vi "Z-trial.vi"() -> ()   [LabVIEW 2010]
panel:
  out "slice number":i32
  out "GetPositionOffset 2":i32
  out "pfPosOffset 2":sgl
  out "pfPosOffset":sgl
  out "GetPositionOffset":i32
  out "pfAbsPos 2":sgl
  out "pfAbsPos":sgl
  out "fAbsPos":sgl
  in  "desired position":dbl
  out "Actual Z position 3":sgl
  in  "move Z absolute value":bool
  out "Actual Z position 2":sgl
  out "GetPosition 2":i32
  in  "get Z":bool
  in  "scan z":bool
  in  "number of slices":i32
  out "Actual Z position":sgl
  out "GetPosition":i32
  out "Cal. Z":dbl
  in  "Z Step Size":dbl
  in  "Starting Z  Position":dbl
  in  "Z scanner":refnum<k7>(container)
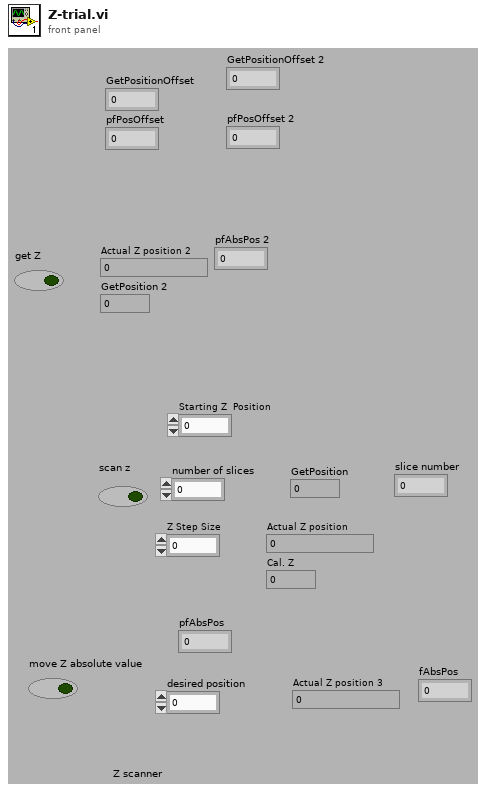
[diagram p1: front panel]
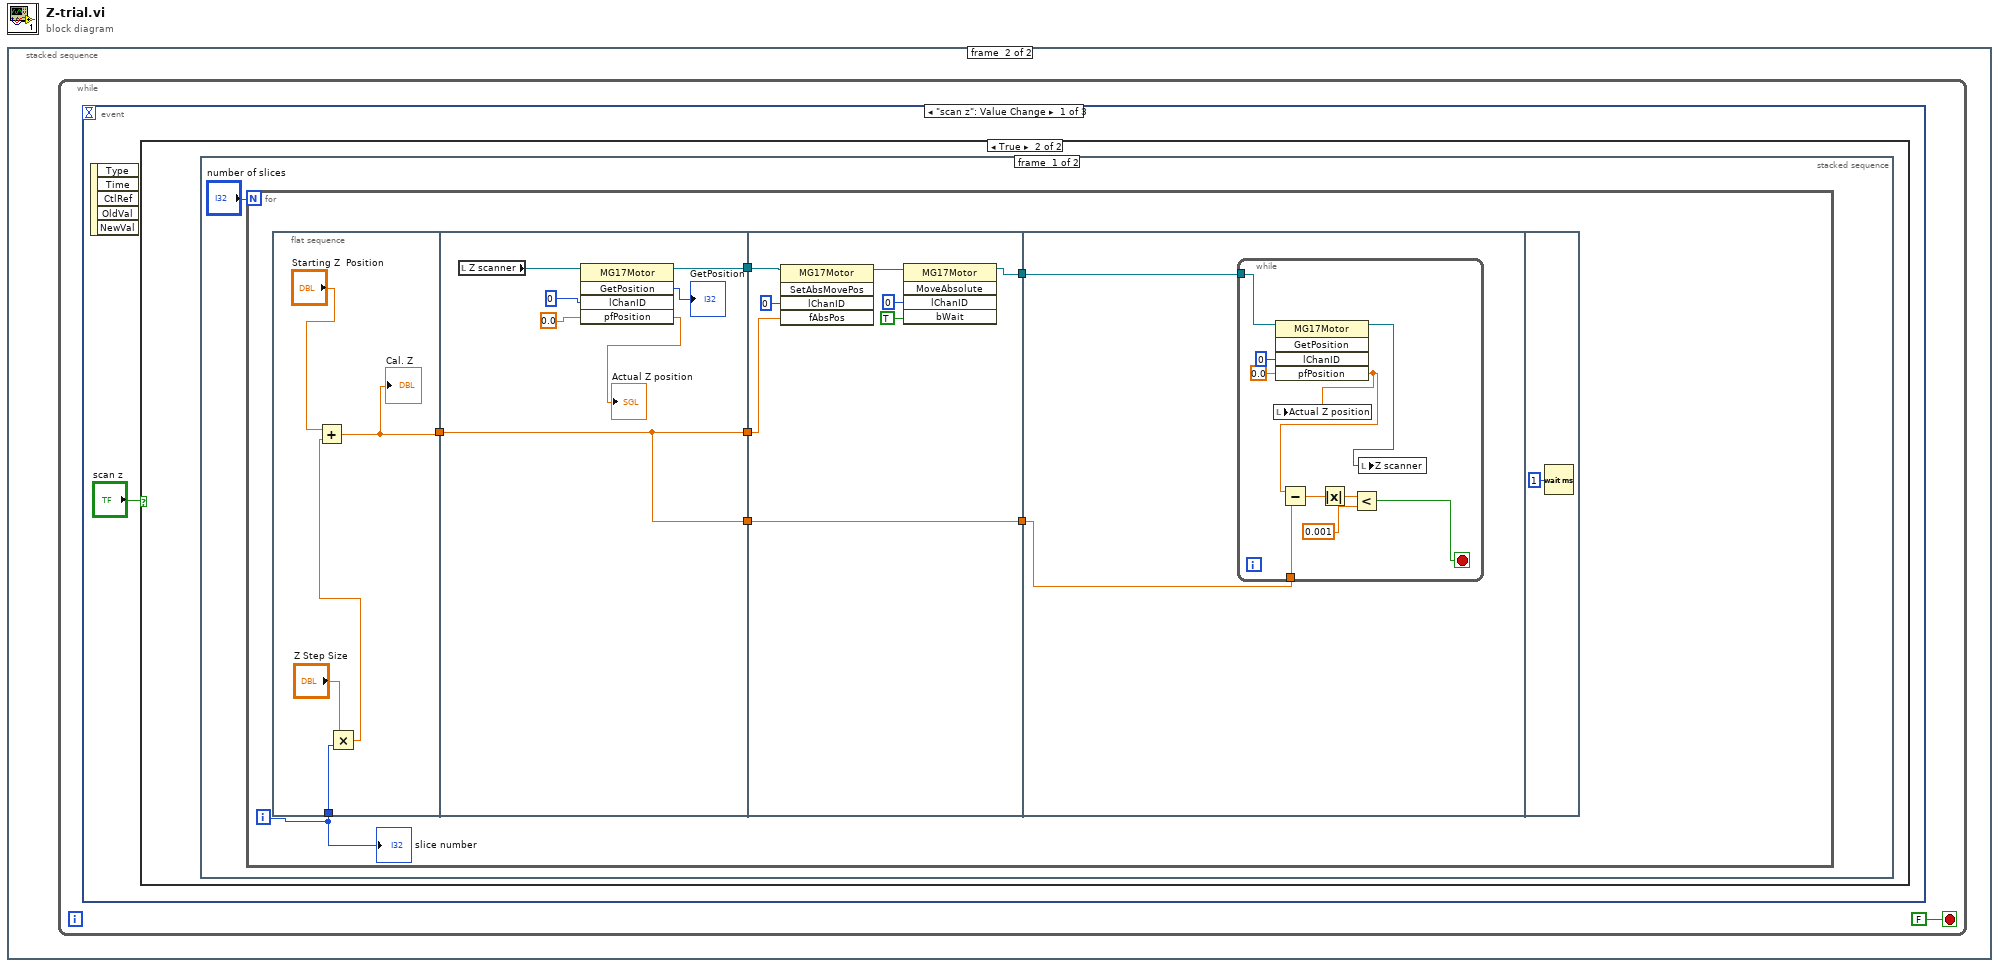
[diagram p0: block diagram]
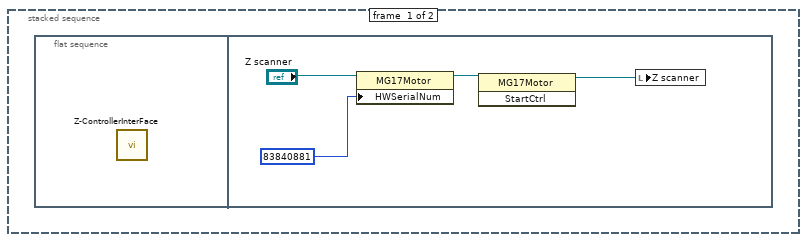
[diagram p2: hidden frame]
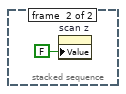
[diagram p4: hidden frame]
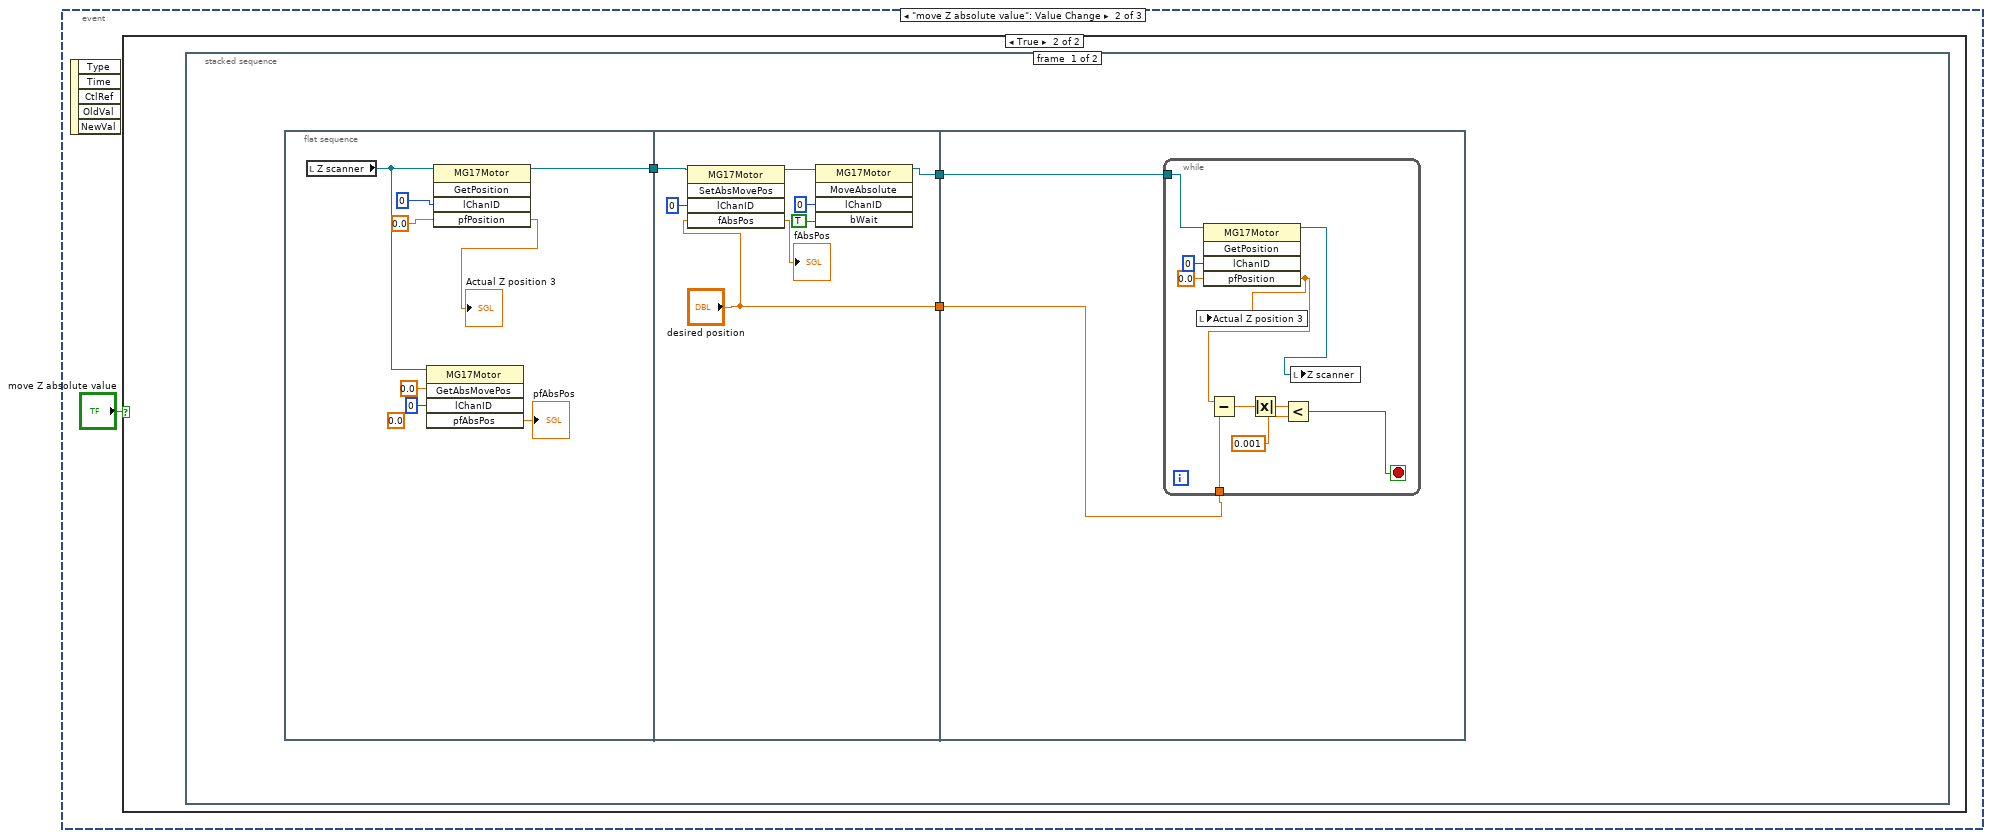
[diagram p5: hidden frame]
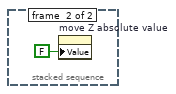
[diagram p7: hidden frame]
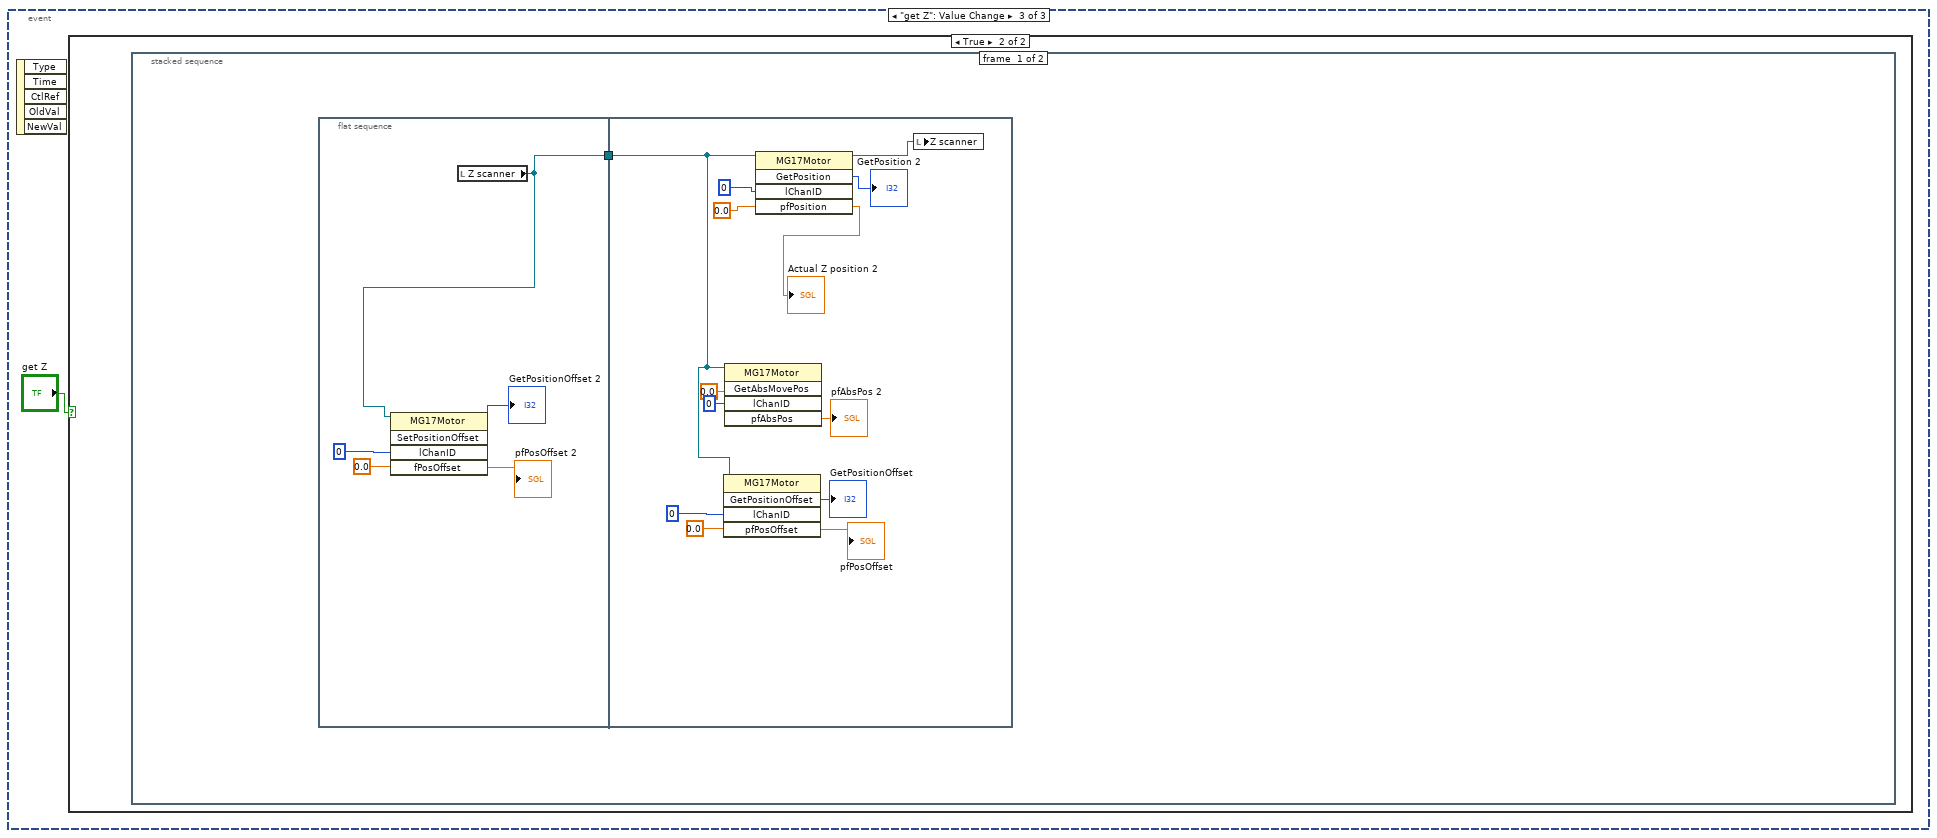
[diagram p8: hidden frame]
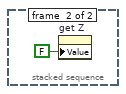
[diagram p10: hidden frame]
diagram:
  n1 = stacked-sequence {
    frame #0 {
      n2 = flat-sequence {
        frame #0 {
          n3 = call "Z-ControllerInterFace.vi"() -> ()  [unwired: 12 in]
        }
        frame #1 {
          n4 = property class="MG17Motor"(reference="Z scanner", "HWSerialNum"=83840881) -> (reference out=w3:refnum<k7>)  [unwired: 1 in, 1 out]
          n5 = invoke class="MG17Motor" method="StartCtrl"(reference=w3) -> (reference out=w1:refnum<k7>)  [unwired: 2 in, 2 out]
          n6 = local write "Z scanner"(w1) -> ()
        }
      }
    }
    frame #1 {
      n7 = while {
        stop <- FALSE stop-if-true
        n8 = event shown="[0] \"scan z\": Value Change" {
          selector: _ -> [_ _ _]
          dyn-events: _ -> [_ _ _]
          timeout: _ -> [_ _ _]
          event "scan z": Value Change {
            n9 = event-data() -> ()  [unwired: 1 in, 5 out]
            n10 = case shown="True" "scan z" {
              frame False {
              }
              frame True {
                n11 = stacked-sequence {
                  frame #0 {
                    n12 = for {
                      N: "number of slices" -> [_]
                      i -> [w8]
                      n13 = flat-sequence {
                        tunnel: [w18] -> w14
                        tunnel: w8 -> [w15]
                        tunnel: [w24] -> w13
                        tunnel: w14 -> [w23]
                        tunnel: [w23] -> w12
                        tunnel: [w23] -> w11
                        tunnel: w13 -> [w34]
                        tunnel: w12 -> [w32]
                        tunnel: w11 -> [w28]
                        tunnel: [w28] -> w10
                        tunnel: [w27] -> w9
                        tunnel: w10 -> [w36]
                        tunnel: w9 -> [w35]
                        frame #0 {
                          n14 = Multiply(x="Z Step Size", y=w15) -> (x*y=w19:dbl)
                          n15 = Add(x="Starting Z  Position", y=w19) -> (x+y=w18:dbl)
                          "Cal. Z" <- w18
                        }
                        frame #1 {
                          n16 = local read "Z scanner"() -> (w22:refnum<k7>)
                          n17 = invoke class="MG17Motor" method="GetPosition"(reference=w22, "lChanID"=0, "pfPosition"=sgl 0.0) -> (reference out=w24:refnum<k7>, "GetPosition"=→"GetPosition":i32, "pfPosition"=→"Actual Z position":sgl)  [unwired: 2 in, 2 out]
                        }
                        frame #2 {
                          n18 = invoke class="MG17Motor" method="SetAbsMovePos"(reference=w34, "lChanID"=0, "fAbsPos"=w32) -> (reference out=w33:refnum<k7>)  [unwired: 2 in, 4 out]
                          n19 = invoke class="MG17Motor" method="MoveAbsolute"(reference=w33, "lChanID"=0, "bWait"=TRUE) -> (reference out=w27:refnum<k7>)  [unwired: 2 in, 4 out]
                        }
                        frame #3 {
                          n20 = while {
                            tunnel: w36 -> [w43]
                            tunnel: w35 -> [w38]
                            stop <- w39 stop-if-true
                            n21 = invoke class="MG17Motor" method="GetPosition"(reference=w38, "lChanID"=0, "pfPosition"=sgl 0.0) -> (reference out=w37:refnum<k7>, "pfPosition"=w44:sgl)  [unwired: 2 in, 3 out]
                            n22 = local write "Actual Z position"(w44) -> ()
                            n23 = Subtract(x=w44, y=w43) -> (x-y=w42:dbl)
                            n24 = Absolute Value(x=w42) -> (abs(x)=w41:dbl)
                            n25 = Less?(x=w41, y=0.001) -> (x < y?=w39:bool)
                            n26 = local write "Z scanner"(w37) -> ()
                          }
                        }
                        frame #4 {
                          n27 = Wait (ms)(milliseconds to wait=u32 1) -> ()  [unwired: 1 out]
                        }
                      }
                      "slice number" <- w8
                    }
                  }
                  frame #1 {
                    n28 = property on="scan z" class="Bool (strict)"("Value"=FALSE ("scan z")) -> ()  [unwired: 2 in, 2 out]
                  }
                }
              }
            }
          }
          event "move Z absolute value": Value Change {
            n29 = event-data() -> ()  [unwired: 1 in, 5 out]
            n30 = case shown="True" "move Z absolute value" {
              frame False {
              }
              frame True {
                n31 = stacked-sequence {
                  frame #0 {
                    n32 = flat-sequence {
                      tunnel: [w58] -> w52
                      tunnel: w52 -> [w68]
                      tunnel: [w63] -> w51
                      tunnel: ["desired position"] -> w50
                      tunnel: w51 -> [w70]
                      tunnel: w50 -> [w69]
                      frame #0 {
                        (unwired) sgl 0.0 ("pfAbsPos")
                        n33 = local read "Z scanner"() -> (w56:refnum<k7>)
                        n34 = invoke class="MG17Motor" method="GetAbsMovePos"(reference=w56, "lChanID"=0, "pfAbsPos"=sgl 0.0) -> ("pfAbsPos"=→"pfAbsPos":sgl)  [unwired: 2 in, 4 out]
                        n35 = invoke class="MG17Motor" method="GetPosition"(reference=w56, "lChanID"=0, "pfPosition"=sgl 0.0) -> (reference out=w58:refnum<k7>, "pfPosition"=→"Actual Z position 3":sgl)  [unwired: 2 in, 3 out]
                      }
                      frame #1 {
                        n36 = invoke class="MG17Motor" method="SetAbsMovePos"(reference=w68, "lChanID"=0, "fAbsPos"="desired position") -> (reference out=w67:refnum<k7>, "fAbsPos"=→"fAbsPos":sgl)  [unwired: 2 in, 3 out]
                        n37 = invoke class="MG17Motor" method="MoveAbsolute"(reference=w67, "lChanID"=0, "bWait"=TRUE) -> (reference out=w63:refnum<k7>)  [unwired: 2 in, 4 out]
                      }
                      frame #2 {
                        n38 = while {
                          tunnel: w69 -> [w77]
                          tunnel: w70 -> [w72]
                          stop <- w73 stop-if-true
                          n39 = invoke class="MG17Motor" method="GetPosition"(reference=w72, "lChanID"=0, "pfPosition"=sgl 0.0) -> (reference out=w71:refnum<k7>, "pfPosition"=w78:sgl)  [unwired: 2 in, 3 out]
                          n40 = local write "Actual Z position 3"(w78) -> ()
                          n41 = Subtract(x=w78, y=w77) -> (x-y=w76:dbl)
                          n42 = Absolute Value(x=w76) -> (abs(x)=w75:dbl)
                          n43 = Less?(x=w75, y=0.001) -> (x < y?=w73:bool)
                          n44 = local write "Z scanner"(w71) -> ()
                        }
                      }
                    }
                  }
                  frame #1 {
                    n45 = property on="move Z absolute value" class="Bool (strict)"("Value"=FALSE ("scan z")) -> ()  [unwired: 2 in, 2 out]
                  }
                }
              }
            }
          }
          event "get Z": Value Change {
            n46 = event-data() -> ()  [unwired: 1 in, 5 out]
            n47 = case shown="True" "get Z" {
              frame False {
              }
              frame True {
                n48 = stacked-sequence {
                  frame #0 {
                    n49 = flat-sequence {
                      tunnel: [w84] -> w83
                      tunnel: w83 -> [w89]
                      frame #0 {
                        n50 = local read "Z scanner"() -> (w84:refnum<k7>)
                        n51 = invoke class="MG17Motor" method="SetPositionOffset"(reference=w84, "lChanID"=0, "fPosOffset"=sgl 0.0 ("pfAbsPos")) -> ("SetPositionOffset"=→"GetPositionOffset 2":i32, "fPosOffset"=→"pfPosOffset 2":sgl)  [unwired: 2 in, 3 out]
                      }
                      frame #1 {
                        n52 = invoke class="MG17Motor" method="GetPositionOffset"(reference=w89, "lChanID"=0, "pfPosOffset"=sgl 0.0 ("pfAbsPos")) -> ("GetPositionOffset"=→"GetPositionOffset":i32, "pfPosOffset"=→"pfPosOffset":sgl)  [unwired: 2 in, 3 out]
                        n53 = invoke class="MG17Motor" method="GetAbsMovePos"(reference=w89, "lChanID"=0, "pfAbsPos"=sgl 0.0) -> ("pfAbsPos"=→"pfAbsPos 2":sgl)  [unwired: 2 in, 4 out]
                        n54 = invoke class="MG17Motor" method="GetPosition"(reference=w89, "lChanID"=0, "pfPosition"=sgl 0.0) -> (reference out=w97:refnum<k7>, "GetPosition"=→"GetPosition 2":i32, "pfPosition"=→"Actual Z position 2":sgl)  [unwired: 2 in, 2 out]
                        n55 = local write "Z scanner"(w97) -> ()
                      }
                    }
                  }
                  frame #1 {
                    n56 = property on="get Z" class="Bool (strict)"("Value"=FALSE ("scan z")) -> ()  [unwired: 2 in, 2 out]
                  }
                }
              }
            }
          }
        }
      }
    }
  }
